vi "MGI For Loop Progress Bar.vi"(4 "Wait Time (ms) (1000)":u32=1000, 5 "Show Time? (T)":bool=TRUE, 6 "Moving Average Size (8)":i32=8, 7 "Total Iter":i32, 8 "error in (no error)":errorcluster, 9 "Allow Abort?(F)":bool caption="Allow Abort? (F)", 10 "Current Iter":i32, 11 "Message":string) -> (0 "error out":errorcluster, 2 "Aborted?":bool)   [LabVIEW 2016]
doc: "This VI is a progress bar for For Loops. If the \"Wait Time\" has elapsed, and the loop is less than half-way through its total # of iterations, this VI will open and show a progress bar for the For Loop.\n\nIf \"Show Time?\" is True, this VI will display an approximation for the time remaining. A moving average is used to smooth the approximation to compensate for non-linearities in code execution.\n\nFreeware from Moore Good Ideas, www.mooregoodideas.com. Do not remove this line."
uses:
  <userlib>/_MGI/1D Array/MGI Running Maximum/MGI Running Maximum (DBL).vi
panel:
  in  "Abort":bool
  out "Time Remaining":dbl format="%#.1t"
  out "Progress Bar":dbl(slide) scale=0.0..1.0
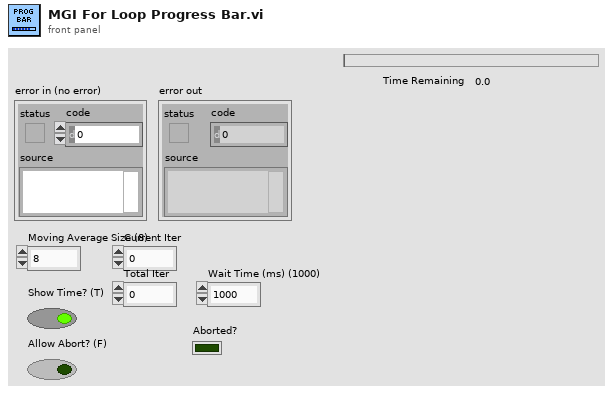
[diagram p1: front panel]
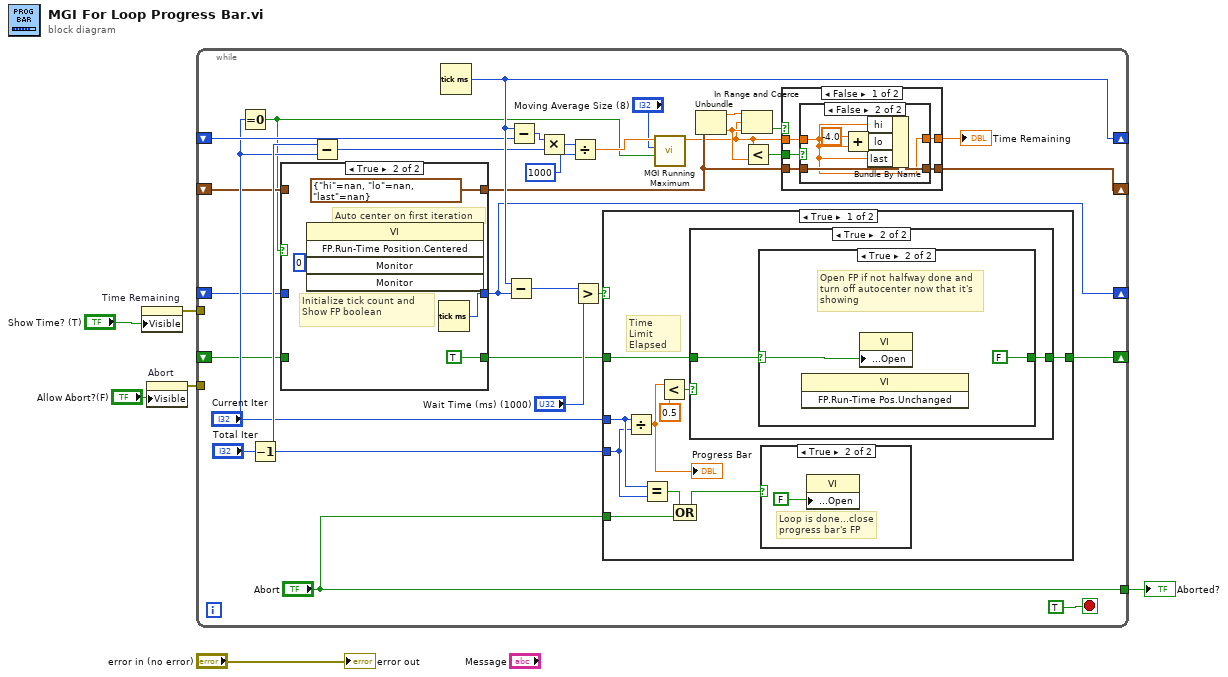
[diagram p0: block diagram]
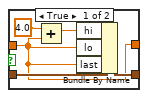
[diagram p2: hidden frame]
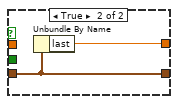
[diagram p3: hidden frame]
diagram:
  n1 = property on="Time Remaining" class="DigNum (strict)"("Visible"="Show Time? (T)") -> (error out=w1:errorcluster)  [unwired: 2 in, 1 out]
  n2 = property on="Abort" class="Bool"("Visible"="Allow Abort?(F)") -> (error out=w4:errorcluster)  [unwired: 2 in, 1 out]
  n3 = while {
    shift-right: [w19] -> _
    shift-left: _ -> [w21]
    shift-right: [w36] -> _
    shift-left: _ -> [w22]
    shift-right: [w35] -> _
    shift-left: _ -> [w34]
    tunnel: ["Abort"] -> w5
    tunnel: w4 -> [_]
    tunnel: w1 -> [_]
    shift-right: [w14] -> _
    shift-left: _ -> [w13]
    stop <- TRUE stop-if-true
    n4 = Equal To 0?(x="Current Iter") -> (x = 0?=w8:bool)
    n5 = Decrement(x="Total Iter") -> (x-1=w28:i32)
    n6 = case shown="True" w8 {
      tunnel: w22 -> [w57 _]
      tunnel: w21 -> [w56 _]
      tunnel: [w57 TRUE] -> w20
      tunnel: [w56 w59] -> w19
      tunnel: [w55 cluster{"hi":dbl, "lo":dbl, "last":dbl} {"hi"=nan, "lo"=nan, "last"=nan}] -> w16
      tunnel: w13 -> [w55 _]
      frame False {
      }
      frame True {
        # "Initialize tick count and Show FP boolean"
        # "Auto center on first iteration"
        n7 = invoke class="VI" method="FP.Run-Time Position.Centered"("Monitor"=i16 0) -> ()  [unwired: 4 in, 5 out]
        n8 = Tick Count (ms)() -> (millisecond timer value=w59:u32)
      }
    }
    n9 = Subtract(x=w28, y="Current Iter") -> (x-y=w32:i32)
    n10 = Tick Count (ms)() -> (millisecond timer value=w35:u32)
    n11 = Subtract(x=w35, y=w19) -> (x-y=w25:u32)
    n12 = Subtract(x=w35, y=w34) -> (x-y=w33:u32)
    n13 = Multiply(x=w33, y=w32) -> (x*y=w31:u32)
    n14 = Divide(x=w31, y=u32 1000 ("x")) -> (x/y=w10:dbl)
    n15 = Greater?(x=w25, y="Wait Time (ms) (1000)") -> (0:w24:bool)
    n16 = case shown="True" w24 {
      tunnel: "Current Iter" -> [w67 _]
      tunnel: w20 -> [w69 w79]
      tunnel: [w68 w79] -> w36
      tunnel: w28 -> [w65 _]
      tunnel: "Abort" -> [w63 _]
      frame True {
        # "Time Limit Elapsed"
        n17 = Divide(x=w67, y=w65) -> (x/y=w66:dbl)
        "Progress Bar" <- w66
        n18 = Equal?(x=w67, y=w65) -> (x = y?=w64:bool)
        n19 = Less?(x=w66, y=0.5) -> (x < y?=w71:bool)
        n20 = Compound Arithmetic op=OR(w64, w63) -> (w62:bool)
        n21 = case shown="True" w71 {
          tunnel: w69 -> [w73 w75]
          tunnel: [w73 w74] -> w68
          frame False {
            # "Progress is over halfway done...just wait it out with no progress bar"
          }
          frame True {
            n22 = case shown="True" w75 {
              selector: w75 -> [w76 w78]
              tunnel: [w76 FALSE] -> w74
              frame False {
                # "FP has already been opened"
              }
              frame True {
                # "Open FP if not halfway done and turn off autocenter now that it's showing"
                n23 = invoke class="VI" method="FP.Run-Time Pos.Unchanged"() -> ()  [unwired: 3 in, 3 out]
                n24 = property class="VI"("Front Panel Window:Open"=w78) -> ()  [unwired: 2 in, 2 out]
              }
            }
          }
        }
        n25 = case shown="True" w62 {
          frame False {
            # "Loop is not done"
          }
          frame True {
            # "Loop is done...close progress bar's FP"
            n26 = property class="VI"("Front Panel Window:Open"=FALSE) -> ()  [unwired: 2 in, 2 out]
          }
        }
      }
      frame False {
        # "Time Limit has not yet elapsed"
      }
    }
    n27 = call-poly <userlib>:"MGI Running Maximum.vi"("Initialize? (F)"=w8, "Size"="Moving Average Size (8)", "Value"=w10) -> ("Maximum"=w7:dbl)  [unwired: 8 in]
    n28 = Unbundle(w16) -> ("hi"=w18:dbl, "last"=w12:dbl)  [unwired: 1 out]
    n29 = In Range and Coerce(upper limit=w18, x=w7, lower limit=w12) -> (In Range?=w17:bool)  [unwired: 1 out]
    n30 = Less?(x=w7, y=w12) -> (x < y?=w11:bool)
    n31 = case shown="False" w17 {
      tunnel: w16 -> [w42 w53]
      tunnel: [w38 w54] -> w15
      tunnel: [w39 w53] -> w14
      tunnel: w11 -> [w41 _]
      tunnel: w7 -> [w40 _]
      frame False {
        n32 = case shown="False" w41 {
          tunnel: w42 -> [w47 w52]
          tunnel: w40 -> [w43 w49]
          tunnel: [w46 w51] -> w39
          tunnel: [w43 w49] -> w38
          frame True {
            n33 = Add(x=4.0 ("Time Remaining"), y=w43) -> (x+y=w45:dbl)
            n34 = Bundle By Name(cluster=w47, "hi"=w45, "lo"=w43, "last"=w43) -> (w46:cluster{"hi":dbl, "lo":dbl, "last":dbl})
          }
          frame False {
            n35 = Add(x=-4.0 ("Time Remaining"), y=w49) -> (x+y=w48:dbl)
            n36 = Bundle By Name(cluster=w52, "hi"=w49, "lo"=w48, "last"=w49) -> (w51:cluster{"hi":dbl, "lo":dbl, "last":dbl})
          }
        }
      }
      frame True {
        n37 = Unbundle By Name(w53) -> ("last"=w54:dbl)
      }
    }
    "Time Remaining" <- w15
  }
  "Aborted?" <- w5
  "error out" <- "error in (no error)"
